vi "Find A Channel.vi"(1 "element":string, 2 "Data Output":T1 {"Data Channels" format="%.2f"}) -> (0 "Signal (V)":dbl[](array[numeric]) format="%.2f")   [LabVIEW 2016, in "impulse functions.lvlib"]
uses:
  impulse functions.lvlib
panel:
  # "Copyright Americo A. Migliaccio (c) 2002 All Rights Reserved by Author"
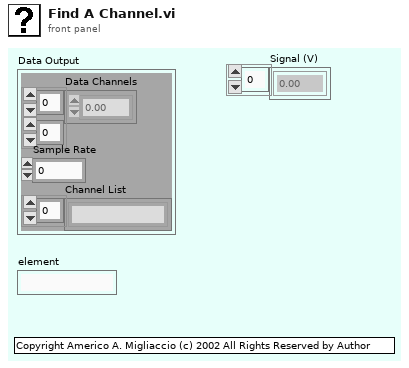
[diagram p1: front panel]
types:
  T1 = cluster{"Data Channels":dbl[][], "Sample Rate":i32, "Channel List":string[]}
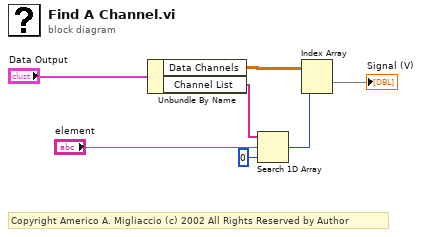
[diagram p0: block diagram]
diagram:
  # "Copyright Americo A. Migliaccio (c) 2002 All Rights Reserved by Author"
  n1 = Unbundle By Name("Data Output") -> ("Data Channels"=w6:dbl[][], "Channel List"=w7:string[])
  n2 = Search 1D Array(1D array=w7, element="element", start index (0)=0) -> (index of element=w3:i32)
  n3 = Index Array(array=w6, index (row)=w3) -> (element=→"Signal (V)":dbl[])  [unwired: 1 in]
